vi "singleTeam.vi"(8 "TeamUniqueID":i32, 9 "Debug":bool, 11 "httpRequestID":u32) -> ()   [LabVIEW 2013]
uses:
  FRCts20_EspEngine.lvlib
  <vilib>/wsapi/NI_WebServices.lvlib
  <vilib>/wsapi/subVIs/Set Boolean ESP Variable.vi
  Web Methods/source/VI Source/Web Method Public Interface/FRCts20_WebMethods_ctl_teamIdentifier.ctl
  Web Methods/source/VI Source/FRCts20_WebMethods.lvlib
  Backend/source/VI Source/FRCts20_Backend_API/FRCts20_Backend_API_SW.ctl
  Backend/source/VI Source/FRCts20_Backend_API/FRCts20_Backend_API.lvlib
  Web Methods/source/VI Source/Web Method Public Interface/FRCts20_WebMethods_ctl_singleTeam.ctl
  Backend/source/VI Source/FRCts20_Backend_API/FRCts20_Backend_API_Status.ctl
  Web Methods/source/VI Source/Web Method Public Interface/FRCts20_WebMethods_ctl_request.ctl
panel:
  in  "Requests":T1[](array[typedef])=[{"Event"="", "Description"="", "Status"=enum."Open", "Open Date"="", "Last Update"="", "Close Date"="", "UniqueId"=0, "Team"={"Team Nickname"="", "Team Number "=0, "UniqueId"=0}, "Comments"=[]}, {"Event"="", "Description"="", "Status"=enum."Open", "Open Date"="", "Last Update"="", "Close Date"="", "UniqueId"=0, "Team"={"Team Nickname"="", "Team Number "=0, "UniqueId"=0}, "Comments"=[]}, {"Event"="", "Description"="", "Status"=enum."Open", "Open Date"="", "Last Update"="", "Close Date"="", "UniqueId"=0, "Team"={"Team Nickname"="", "Team Number "=0, "UniqueId"=0}, "Comments"=[]}]
  in  "Team":T3={"Events"=["New York City"], "Robot Name"="", "Kinect"=TRUE, "Vision"=TRUE, "Can"=FALSE, "Tags"="", "Avatar URL"="http://upload.wikimedia.org/wikipedia/commons/thumb/e/e1/FullMoon2010.jpg/280px-FullMoon2010.jpg", "Team"={"Team Nickname"="Robobunnies", "Team Number "=99, "UniqueId"=1099}, "SWType"="LabVIEW"}
  out "error out":errorcluster
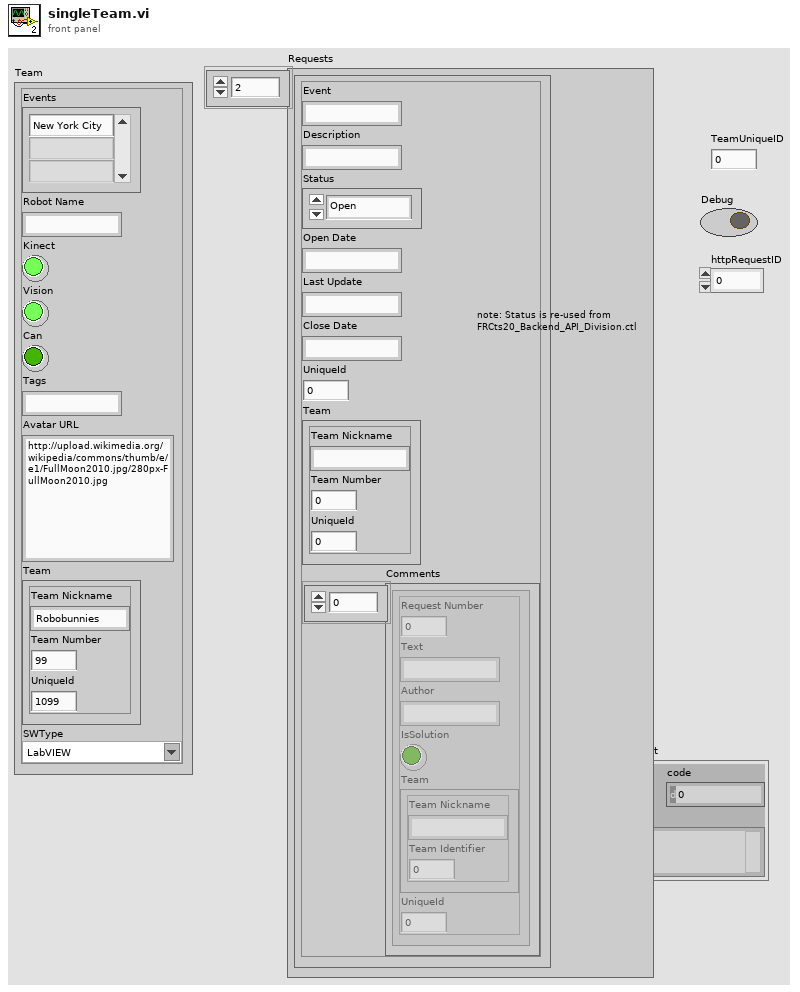
[diagram p1: front panel]
types:
  T1 = typedef "FRCts20_WebMethods.lvlib/FRCts20_WebMethods_ctl_request.ctl" = cluster{"Event":string, "Description":string, "Status":T2, "Open Date":string, "Last Update":string, "Close Date":string, "UniqueId":i32, "Team":cluster{"Team Nickname":string, "Team Number ":i32, "UniqueId":i32}, "Comments":cluster{"Request Number":dbl, "Text":string, "Author":string, "IsSolution":bool, "Team":cluster{"Team Nickname":string, "Team Identifier ":dbl}, "UniqueId":i32}[]}
  T2 = typedef "FRCts20_Backend_API.lvlib/FRCts20_Backend_API_Status.ctl" = enum16{"Open", "In Work", "Closed"}
  T3 = typedef "FRCts20_WebMethods.lvlib/FRCts20_WebMethods_ctl_singleTeam.ctl" = cluster{"Events":string[], "Robot Name":string, "Kinect":bool, "Vision":bool, "Can":bool, "Tags":string, "Avatar URL":string, "Team":T4, "SWType":T5}
  T4 = typedef "FRCts20_WebMethods.lvlib/FRCts20_WebMethods_ctl_teamIdentifier.ctl" = cluster{"Team Nickname":string, "Team Number ":u32, "UniqueId":u32}
  T5 = typedef "FRCts20_Backend_API.lvlib/FRCts20_Backend_API_SW.ctl" = string
  T6 = typedef "FRCts20_EspEngine.lvlib/FRCts20_EspEngine_SearchBrowser.ctl" = cluster{"Event":cluster{"Event Index":u32, "Event Name":string, "Start Time":timestamp, "End Time":timestamp, "OpenIssues":u8, "IsLive":bool}[], "select-choice-software":string, "select-choice-location":string}
  T7 = typedef "FRCts20_EspEngine.lvlib/FRCts20_EspEngine_Team.ctl" = cluster{"Team":T3, "RequestListLength":i16, "Requests":T1[]}
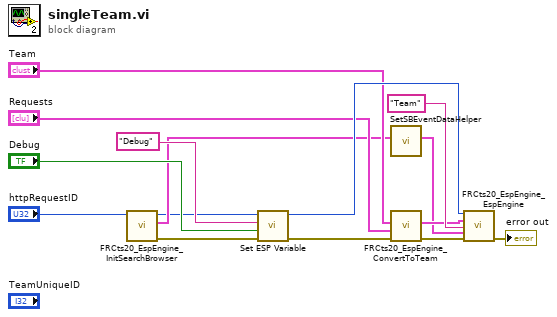
[diagram p0: block diagram]
diagram:
  n1 = call "FRCts20_EspEngine_InitSearchBrowser.vi"("httpRequestID"="httpRequestID") -> ("error out"=w3:errorcluster, "SearchBrowser"=w5:T6, "httpRequestID out"=w1:u32)  [unwired: 8 in]
  n2 = call-poly <vilib>:"Set ESP Variable.vi"("error in (no error)"=w3, "value"="Debug", "key"="Debug", "httpRequestID"=w1) -> ("error out"=w7:errorcluster, "httpRequestID out"=w13:u32)  [unwired: 6 in]
  n3 = call "SetSBEventDataHelper.vi"("SearchBrowser"=w5) -> ("SearchBrowser"=w4:T6)  [unwired: 10 in]
  n4 = call "FRCts20_EspEngine_ConvertToTeam.vi"("error in (no error)"=w7, "Requests"="Requests", "Team"="Team") -> ("error out"=w6:errorcluster, "Team"=w9:T7)  [unwired: 7 in]
  n5 = call "FRCts20_EspEngine_EspEngine.vi"("httpRequestID"=w13, "Cluster"=w9, "Page"="Team", "SearchBrowser"=w4, "error in (no error)"=w6) -> ("error out"=→"error out":errorcluster)  [unwired: 9 in, 1 out]
